vi "Extract Legacy Fields.vi"(9 "Checked Tokens in":cluster{"token type":T4, T2}[](array[cluster]), 10 "JSON Object Descriptor":T1, 11 "source in":string) -> (1 "source out":string, 2 "code":i32, 3 "status":bool)   [LabVIEW 2020, in "Multi Error Cluster.lvlib"]
doc: "Extract the status, code, and source from a tokenized error cluster."
uses:
  <vilib>/MultiError/TokenizeJSON/Multi Error Cluster.lvlib
  <vilib>/MultiError/TokenizeJSON/JSON Token Values.ctl
  <vilib>/MultiError/Errors Cluster Multiple Errors/JSON Token Descriptor.ctl
  <vilib>/MultiError/TokenizeJSON/JSON Raw Token Values.ctl
  <vilib>/MultiError/Errors Cluster Multiple Errors/JSON Object Descriptor.ctl
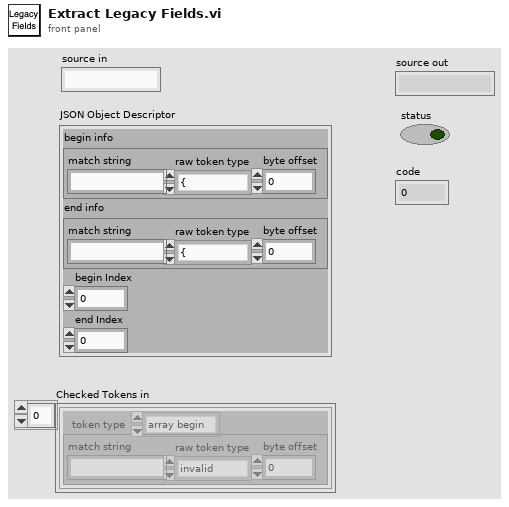
[diagram p1: front panel]
types:
  T1 = typedef "Multi Error Cluster.lvlib/JSON Object Descriptor.ctl" = cluster{"begin info":T2, "end info":T2, "begin Index":i32, "end Index":i32}
  T2 = typedef "Multi Error Cluster.lvlib/JSON Token Descriptor.ctl" = cluster{"match string":string, "raw token type":T3, "byte offset ":i32}
  T3 = typedef "Multi Error Cluster.lvlib/JSON Raw Token Values.ctl" = enum32{"{", "}", "[", "]", ",", ":", "\"", "number", "string", "true", "false", "null", "invalid"}
  T4 = typedef "Multi Error Cluster.lvlib/JSON Token Values.ctl" = enum32{"array begin", "array end", "object begin", "object end", "value", "invalid", "name"}
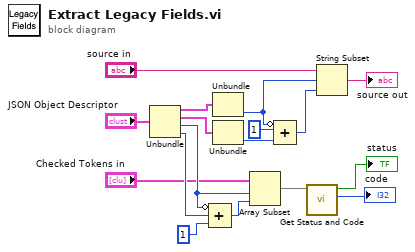
[diagram p0: block diagram]
diagram:
  n1 = Unbundle("JSON Object Descriptor") -> ("begin info"=w2:T2, "end info"=w3:T2, "begin Index"=w10:i32, "end Index"=w11:i32)
  n2 = Compound Arithmetic op=ADD(invert w10, w11, 1) -> (w9:i32)
  n3 = Unbundle(w2) -> ("byte offset"=w6:i32)  [unwired: 2 out]
  n4 = Unbundle(w3) -> ("byte offset"=w4:i32)  [unwired: 2 out]
  n5 = Array Subset(array="Checked Tokens in", index=w10, length=w9) -> (w12:cluster{"token type":T4, T2}[])
  n6 = Compound Arithmetic op=ADD(invert w6, 1, w4) -> (w5:i32)
  n7 = call <vilib>:"Get Status and Code.vi"("tokens"=w12) -> ("code"=→"code":i32, "status"=→"status":bool)  [unwired: 6 in, 3 out]
  n8 = String Subset(string="source in", offset (0)=w6, length (rest)=w5) -> (substring=→"source out":string)
